vi "erForceRobotCommand.vi"(8 "error in (no error)":errorcluster, 10 "robot":T1, 11 "Communication in":refnum<class "Communication.lvclass">) -> (0 "error out":errorcluster, 2 "robotCommandArray out":u8[](array[numeric]), 3 "Communication out":refnum<class "Communication.lvclass">)   [LabVIEW 2023, in "Communication.lvclass"]
uses:
  Communication.lvclass
  Convert AI Robot to Robot Command Folder/grSim/grSim Robot Command.ctl
  MessageAI_State Folder/Varint Encoder uint32.vi
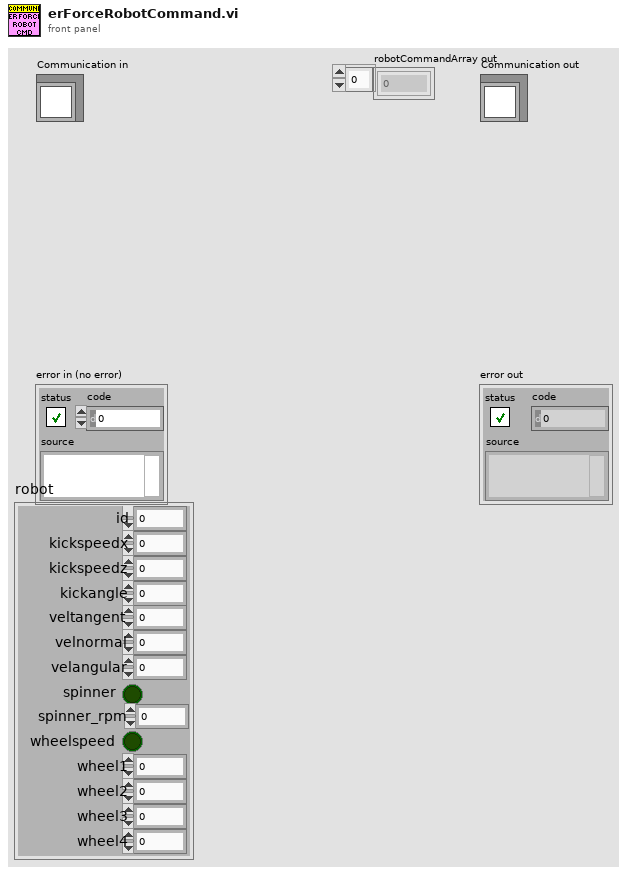
[diagram p1: front panel]
types:
  T1 = typedef "grSim Robot Command.ctl" = cluster{"id":u32, "kickspeedx":sgl, "kickspeedz":sgl, "veltangent":sgl, "velnormal":sgl, "velangular":sgl, "spinner":bool, "wheelspeed":bool, "wheel1":sgl, "wheel2":sgl, "wheel3":sgl, "wheel4":sgl, "kickangle":sgl, "spinner_rpm":sgl}
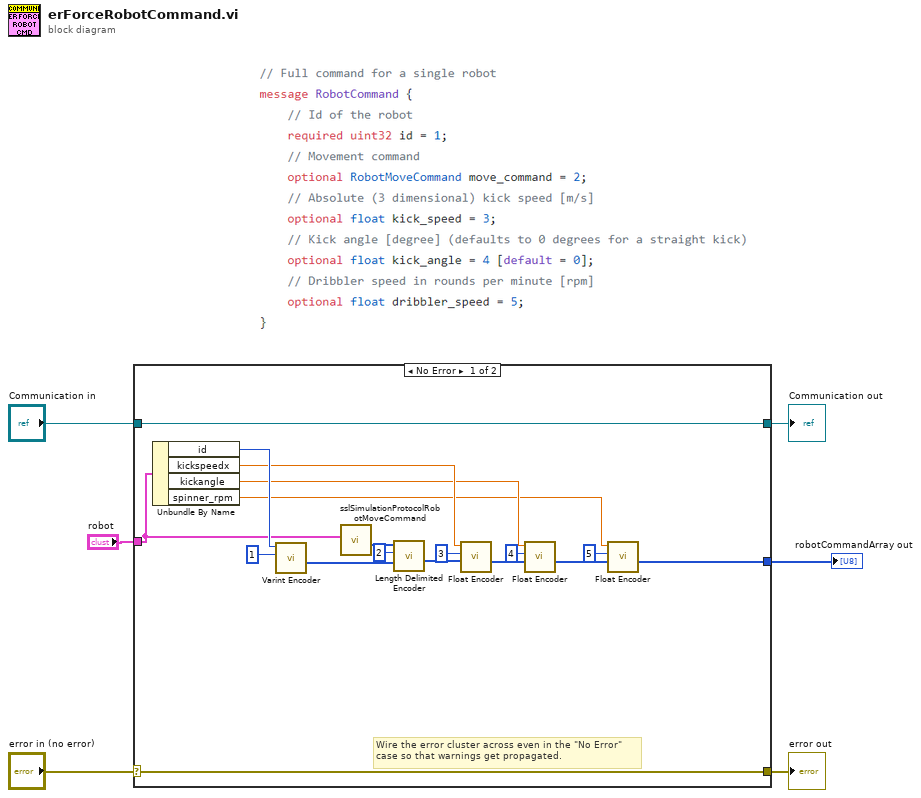
[diagram p0: block diagram]
diagram:
  n1 = case shown="No Error" "error in (no error)" {
    selector: "error in (no error)" -> [w23 w26]
    tunnel: [w23 w26] -> w5
    tunnel: [w24 w25] -> w3
    tunnel: "Communication in" -> [w24 w25]
    tunnel: [w16 _] -> w2
    tunnel: "robot" -> [w8 _]
    frame No Error {
      # "Wire the error cluster across even in the \"No Error\"\ncase so that warnings get propagated."
      n2 = Unbundle By Name(w8) -> ("id"=w12:u32, "kickspeedx"=w11:sgl, "kickangle"=w10:sgl, "spinner_rpm"=w9:sgl)
      n3 = call-poly "Varint Encoder.vi"("Key"=u32 1, "Value"=w12) -> ("Array"=w7:u8[])  [unwired: 9 in]
      n4 = call "sslSimulationProtocolRobotMoveCommand.vi"("robot"=w8) -> ("robotMoveCommand"=w15:u8[])  [unwired: 8 in, 2 out]
      n5 = call "Length Delimited Encoder.vi"("Original Array In"=w7, "Key"=u32 2, "Array In to be added"=w15) -> ("Array"=w13:u8[])  [unwired: 8 in]
      n6 = call "Float Encoder.vi"("Array In"=w13, "Key"=u32 3, "Value"=w11) -> ("Array"=w19:u8[])  [unwired: 8 in]
      n7 = call "Float Encoder.vi"("Array In"=w19, "Key"=u32 4, "Value"=w10) -> ("Array"=w17:u8[])  [unwired: 8 in]
      n8 = call "Float Encoder.vi"("Array In"=w17, "Key"=u32 5, "Value"=w9) -> ("Array"=w16:u8[])  [unwired: 8 in]
    }
    frame Error {
    }
  }
  "error out" <- w5
  "Communication out" <- w3
  "robotCommandArray out" <- w2
